vi "API_Sample Data Notifier Constant.vi"() -> (3 "Sample Data Notifier":refnum<notifier>)   [LabVIEW 2015, in "Tool Module.lvlib"]
doc: "Provides a Sample data Notifier Constant for initialization, if needed in Host app."
uses:
  Tool Module.lvlib
  Support/_Sample Data Rtn Cluster--typedef.ctl
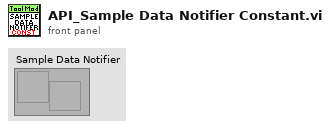
[diagram p1: front panel]
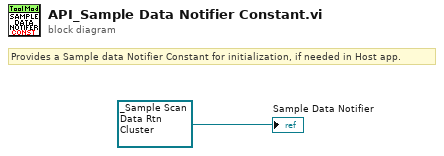
[diagram p0: block diagram]
diagram:
  # "Provides a Sample data Notifier Constant for initialization, if needed in Host app."
  "Sample Data Notifier" <- refnum<notifier> refnum ("Sample Data Notifier")
